vi "Write voltage range.vi"(8 "error in (no error)":errorcluster caption="에러 입력(에러 없음)", 10 "voltage range":dbl, 11 "Waveform Obj 입력":refnum<class "Waveform Obj.lvclass">) -> (0 "error out":errorcluster caption="에러 출력", 3 "Waveform Obj 출력":refnum<class "Waveform Obj.lvclass">)   [LabVIEW 2020, in "Waveform Obj.lvclass"]
uses:
  Waveform Obj.lvclass
  Waveform Obj.lvclass/Waveform Obj.ctl
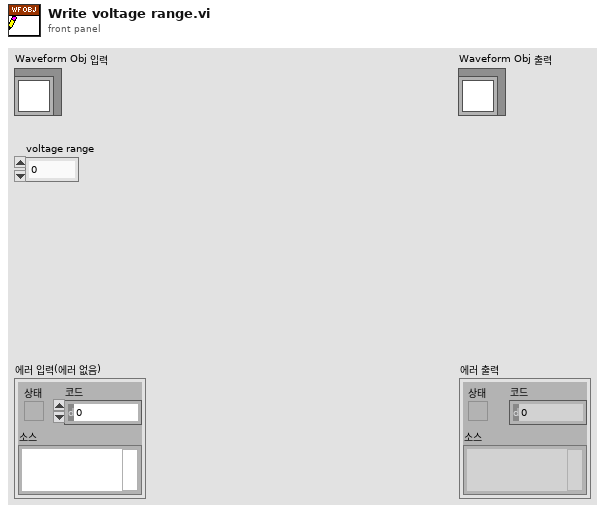
[diagram p1: front panel]
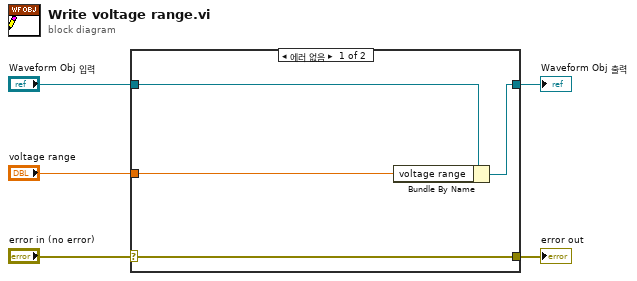
[diagram p0: block diagram]
diagram:
  n1 = case shown="에러 없음" "error in (no error)" {
    selector: "error in (no error)" -> [w9 w10]
    tunnel: [w9 w10] -> w4
    tunnel: [w7 w11] -> w2
    tunnel: "Waveform Obj 입력" -> [w8 w11]
    tunnel: "voltage range" -> [w6 _]
    frame No Error {
      n2 = Bundle By Name(cluster=w8, "voltage range"=w6) -> (w7:refnum<class "Waveform Obj.lvclass">)
    }
    frame Error {
    }
  }
  "error out" <- w4
  "Waveform Obj 출력" <- w2
